vi "Create From Variant.vi"(8 "error in (no error)":errorcluster, 10 "Variant":variant, 11 "JSON Null in":refnum<class "JSON Null.lvclass">) -> (0 "error out":errorcluster, 3 "JSON Null out":refnum<class "JSON Null.lvclass">)   [LabVIEW 2015, in "LVJSON.lvlib" / "JSON Null.lvclass"]
uses:
  JSON Null.lvclass
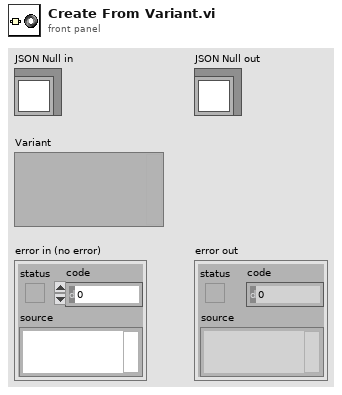
[diagram p1: front panel]
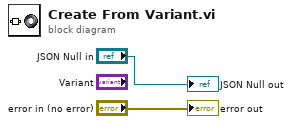
[diagram p0: block diagram]
diagram:
  "error out" <- "error in (no error)"
  "JSON Null out" <- "JSON Null in"
